vi "VCS Get Ec Motor Parameter.vi"(4 "error in (no error)":errorcluster, 7 "axis in":cluster{"keyHandle":u32, "nodeId":u16}={"keyHandle"=0, "nodeId"=1}) -> (0 "error out":errorcluster, 1 "EC motor parameter":T1, 3 "axis out":cluster{"keyHandle":u32, "nodeId":u16}={"keyHandle"=0, "nodeId"=1})   [LabVIEW 2018]
doc: "With function <B>VCS_GetEcMotorParameter<B></B> it is possible to read all EC motor parameters."
uses:
  Resources/EposCmd.dll
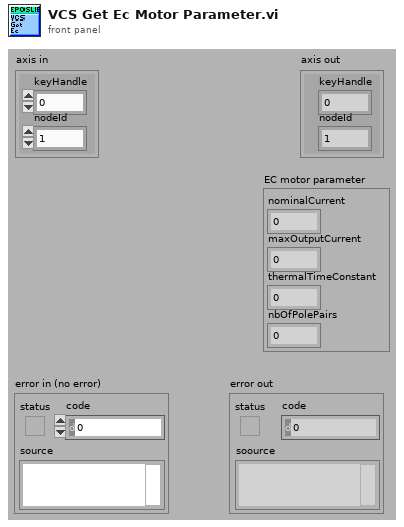
[diagram p1: front panel]
types:
  T1 = cluster{"nominalCurrent":u16, "maxOutputCurrent":u16, "thermalTimeConstant":u16, "nbOfPolePairs":u8}
  T2 = cluster{"pNominalCurrent":u16, "pMaxOutputCurrent":u16, "pThermalTimeConstant":u16, "pNbOfPolePairs":u8}
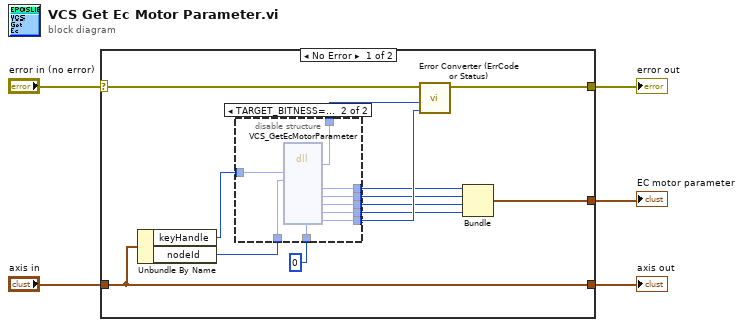
[diagram p0: block diagram]
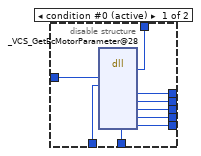
[diagram p2: hidden frame]
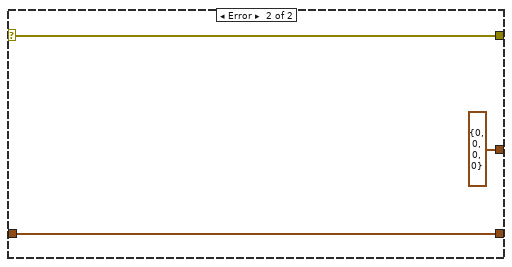
[diagram p3: hidden frame]
diagram:
  n1 = case shown="No Error" "error in (no error)" {
    selector: "error in (no error)" -> [w16 w38]
    tunnel: "axis in" -> [w18 w39]
    tunnel: [w18 w39] -> w4
    tunnel: [w17 w38] -> w3
    tunnel: [w6 T2 {"pNominalCurrent"=0, "pMaxOutputCurrent"=0, "pThermalTimeConstant"=0, "pNbOfPolePairs"=0}] -> w1
    frame No Error {
      n2 = Unbundle By Name(w18) -> ("keyHandle"=w15:u32, "nodeId"=w14:u16)
      n3 = disable-structure shown="TARGET_BITNESS==64" {
        disable-tunnel: w15 -> [w27 w36]
        disable-tunnel: w14 -> [w26 w35]
        disable-tunnel: u32 0 ("pErrorCode") -> [w25 w34]
        disable-tunnel: [w24 w33] -> w12
        disable-tunnel: [w23 w32] -> w11
        disable-tunnel: [w22 w31] -> w10
        disable-tunnel: [w21 w30] -> w9
        disable-tunnel: [w20 w29] -> w8
        disable-tunnel: [w19 w28] -> w7
        frame condition #0 (active) {
          n4 = dll-call lib="C:/Projeto em LabVIEW/EPOS-LabVIEW-Instrument-Driver-En/LabVIEW/maxon EPOS/Resources/EposCmd.*" fn="_VCS_GetEcMotorParameter@28"("KeyHandle"=w27, "NodeId"=w26, "pErrorCode"=w25) -> ("Rückgabetyp"=w24:i32, "pNominalCurrent"=w22:u16, "pMaxOutputCurrent"=w21:u16, "pThermalTimeConstant"=w19:u16, "pNbOfPolePairs"=w20:u8, "pErrorCode"=w23:u32)  [unwired: 9 in, 2 out]
        }
        frame condition #1 {
          n5 = dll-call lib="C:/Projeto em LabVIEW/EPOS-LabVIEW-Instrument-Driver-En/LabVIEW/maxon EPOS/Resources/EposCmd.dll" fn="VCS_GetEcMotorParameter" ("EposCmd.dll:_VCS_GetEcMotorParameter@28")("KeyHandle"=w36, "NodeId"=w35, "pErrorCode"=w34) -> ("Rückgabetyp"=w33:i32, "pNominalCurrent"=w31:u16, "pMaxOutputCurrent"=w30:u16, "pThermalTimeConstant"=w28:u16, "pNbOfPolePairs"=w29:u8, "pErrorCode"=w32:u32)  [unwired: 9 in, 2 out]
        }
      }
      n6 = call "Error Converter (ErrCode or Status).vi"("error code"=w11, "return type"=w12, "error in (no error)"=w16) -> ("error out"=w17:errorcluster)  [unwired: 7 in]
      n7 = Bundle("pNominalCurrent"=w10, "pMaxOutputCurrent"=w9, "pThermalTimeConstant"=w7, "pNbOfPolePairs"=w8) -> (w6:T2)  [unwired: 1 in]
    }
    frame Error {
    }
  }
  "error out" <- w3
  "axis out" <- w4
  "EC motor parameter" <- w1
